vi "BRig_RT__Case_Exp__storeData__endExp__v4.vi"(0 "input_dataBlock":dbl[][](array[numeric]), 1 "input_dataCurrent":dbl[](array[numeric]), 2 "input_dataLick":dbl[][](array[numeric]), 3 "input_dataLC":dbl[](array[numeric]), 4 "input_dataExp":dbl[](array[numeric]), 5 "input_dataTrial":dbl[][](array[numeric]), 7 "input_dataExp_end":dbl[](array[numeric]), 9 "input_dataLC_end":dbl[](array[numeric]), 11 "input_dataMTrig":dbl[](array[numeric]), 12 "input_dataAnalog_trimmed":dbl[][](array[numeric])) -> ()   [LabVIEW 2014]
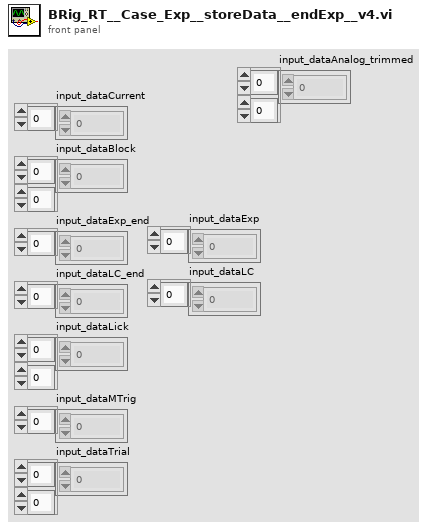
[diagram p1: front panel]
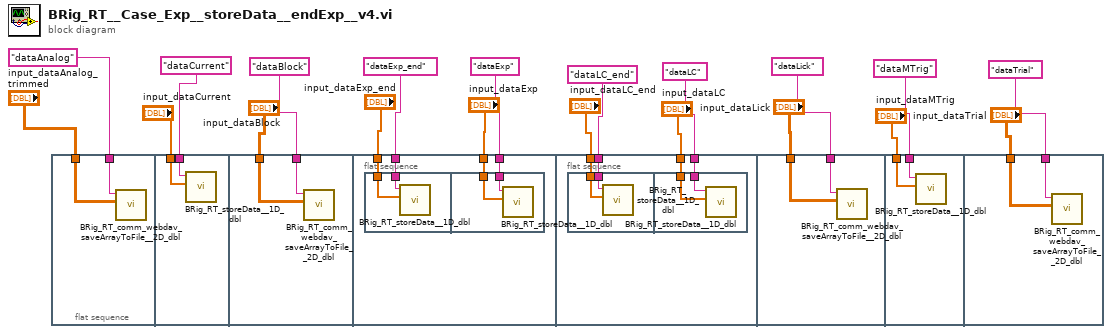
[diagram p0: block diagram]
diagram:
  n1 = flat-sequence {
    tunnel: "input_dataAnalog_trimmed" -> [w21]
    tunnel: "dataAnalog" ("input_filename") -> [w22]
    tunnel: "dataCurrent" ("input_filename") -> [w24]
    tunnel: "input_dataCurrent" -> [w23]
    tunnel: "input_dataBlock" -> [w25]
    tunnel: "dataBlock" ("input_filename") -> [w26]
    tunnel: "input_dataExp_end" -> [w30]
    tunnel: "dataExp_end" ("input_filename") -> [w29]
    tunnel: "input_dataExp" -> [w28]
    tunnel: "dataExp" ("input_filename") -> [w27]
    tunnel: "input_dataLC_end" -> [w38]
    tunnel: "dataLC_end" ("input_filename") -> [w37]
    tunnel: "dataLC" ("input_filename") -> [w36]
    tunnel: "input_dataLC" -> [w35]
    tunnel: "input_dataLick" -> [w43]
    tunnel: "dataLick" ("input_filename") -> [w44]
    tunnel: "input_dataMTrig" -> [w46]
    tunnel: "dataMTrig" ("input_filename") -> [w45]
    tunnel: "input_dataTrial" -> [w47]
    tunnel: "dataTrial" ("input_filename") -> [w48]
    frame #0 {
      n2 = call "BRig_RT_comm_webdav_saveArrayToFile__2D_dbl.vi"("Array"=w21, "input_filename"=w22) -> ()  [unwired: 10 in]
    }
    frame #1 {
      n3 = call "BRig_RT_storeData__1D_dbl.vi"("Array"=w23, "input_filename"=w24) -> ()  [unwired: 10 in]
    }
    frame #2 {
      n4 = call "BRig_RT_comm_webdav_saveArrayToFile__2D_dbl.vi"("Array"=w25, "input_filename"=w26) -> ()  [unwired: 10 in]
    }
    frame #3 {
      n5 = flat-sequence {
        tunnel: w30 -> [w32]
        tunnel: w29 -> [w31]
        tunnel: w28 -> [w33]
        tunnel: w27 -> [w34]
        frame #0 {
          n6 = call "BRig_RT_storeData__1D_dbl.vi"("Array"=w32, "input_filename"=w31) -> ()  [unwired: 10 in]
        }
        frame #1 {
          n7 = call "BRig_RT_storeData__1D_dbl.vi"("Array"=w33, "input_filename"=w34) -> ()  [unwired: 10 in]
        }
      }
    }
    frame #4 {
      n8 = flat-sequence {
        tunnel: w38 -> [w40]
        tunnel: w37 -> [w39]
        tunnel: w36 -> [w42]
        tunnel: w35 -> [w41]
        frame #0 {
          n9 = call "BRig_RT_storeData__1D_dbl.vi"("Array"=w40, "input_filename"=w39) -> ()  [unwired: 10 in]
        }
        frame #1 {
          n10 = call "BRig_RT_storeData__1D_dbl.vi"("Array"=w41, "input_filename"=w42) -> ()  [unwired: 10 in]
        }
      }
    }
    frame #5 {
      n11 = call "BRig_RT_comm_webdav_saveArrayToFile__2D_dbl.vi"("Array"=w43, "input_filename"=w44) -> ()  [unwired: 10 in]
    }
    frame #6 {
      n12 = call "BRig_RT_storeData__1D_dbl.vi"("Array"=w46, "input_filename"=w45) -> ()  [unwired: 10 in]
    }
    frame #7 {
      n13 = call "BRig_RT_comm_webdav_saveArrayToFile__2D_dbl.vi"("Array"=w47, "input_filename"=w48) -> ()  [unwired: 10 in]
    }
  }
